vi "Lab Panel V4.86.vi"() -> ()   [LabVIEW 2013] (continued)
                      frame True {
                      }
                    }
                    n1931 = Unbundle By Name(w3326) -> ("1  (A) cal"=w3319:dbl, "1 (V) cal"=w3318:dbl, "1 (PF) cal"=w3317:dbl, "2 (A) cal"=w3316:dbl, "2 (V) cal"=w3315:dbl, "2 (PF) cal"=w3314:dbl)  [unwired: 4 out]
                    n1932 = Multiply(x=w3325, y=w3319) -> (x*y=w3312:dbl)
                    n1933 = Multiply(x=w3324, y=w3318) -> (x*y=w3311:dbl)
                    n1934 = Multiply(x=w3323, y=w3317) -> (x*y=w3310:dbl)
                    n1935 = Multiply(x=w3322, y=w3316) -> (x*y=w3308:dbl)
                    n1936 = Multiply(x=w3321, y=w3315) -> (x*y=w3307:dbl)
                    n1937 = Multiply(x=w3320, y=w3314) -> (x*y=w3306:dbl)
                    n1938 = local read "SIG LAB04-1"() -> (w3313:T2)
                    n1939 = local read "SIG LAB04-2"() -> (w3309:T2)
                    n1940 = Bundle By Name(cluster=w3313, "AMPS"=w3312, "VOLTS"=w3311, "PF"=w3310) -> (w3302:T2)
                    n1941 = Bundle By Name(cluster=w3309, "AMPS"=w3308, "VOLTS"=w3307, "PF"=w3306) -> (w3301:T2)
                    n1942 = global write "Global display 1.vi" "SIG LAB04-2"(w3301) -> ()
                    n1943 = global write "Global display 1.vi" "SIG LAB04-1"(w3302) -> ()
                    n1944 = local write "SIG LAB04-2"(w3301) -> ()
                    n1945 = local write "SIG LAB04-1"(w3302) -> ()
                  }
                  frame #5 {
                    n1946 = Unbundle By Name(w3334) -> ("LAB05-1 (A)"=w3353:dbl, "LAB05-1 (V)"=w3333:dbl, "LAB05-1 (PF)"=w3352:dbl, "LAB05-2 (A)"=w3351:dbl, "LAB05-2 (V)"=w3350:dbl, "LAB05-2 (PF)"=w3349:dbl)
                    n1947 = case shown="False" w3332 {
                      tunnel: [w3355 w3356] -> w3354
                      tunnel: w3331 -> [_ w3356]
                      frame False {
                        n1948 = local read "CAL LAB05"() -> (w3355:T12)
                      }
                      frame True {
                      }
                    }
                    n1949 = Unbundle By Name(w3354) -> ("1  (A) cal"=w3348:dbl, "1 (V) cal"=w3347:dbl, "1 (PF) cal"=w3346:dbl, "2 (A) cal"=w3345:dbl, "2 (V) cal"=w3344:dbl, "2 (PF) cal"=w3343:dbl)  [unwired: 4 out]
                    n1950 = Multiply(x=w3353, y=w3348) -> (x*y=w3341:dbl)
                    n1951 = Multiply(x=w3333, y=w3347) -> (x*y=w3340:dbl)
                    n1952 = Multiply(x=w3352, y=w3346) -> (x*y=w3339:dbl)
                    n1953 = Multiply(x=w3351, y=w3345) -> (x*y=w3337:dbl)
                    n1954 = Multiply(x=w3350, y=w3344) -> (x*y=w3336:dbl)
                    n1955 = Multiply(x=w3349, y=w3343) -> (x*y=w3335:dbl)
                    n1956 = local read "SIG LAB05-1"() -> (w3342:T2)
                    n1957 = local read "SIG LAB05-2"() -> (w3338:T2)
                    n1958 = Bundle By Name(cluster=w3342, "AMPS"=w3341, "VOLTS"=w3340, "PF"=w3339) -> (w3330:T2)
                    n1959 = Bundle By Name(cluster=w3338, "AMPS"=w3337, "VOLTS"=w3336, "PF"=w3335) -> (w3329:T2)
                    n1960 = global write "Global display 1.vi" "SIG LAB05-1"(w3330) -> ()
                    n1961 = global write "Global display 1.vi" "SIG LAB05-2"(w3329) -> ()
                    n1962 = local write "SIG LAB05-2"(w3329) -> ()
                    n1963 = local write "SIG LAB05-1"(w3330) -> ()
                  }
                }
              }
            }
          }
          frame #12 {
            # "save test data to file"
            n1964 = Get Date/Time In Seconds() -> (seconds since 1Jan1904=w3357:timestamp)
            "File Time Stamp" <- w3357
            n1965 = local read "on loops"() -> (w3376:dbl)
            n1966 = local read "jig cycle"() -> (w3373:dbl)
            n1967 = Format Date/Time String(time format string (%c)="%H:%M%:%S", seconds (now)=w3357) -> (date/time string=w3361:string)  [unwired: 1 in]
            n1968 = Add(x=w3376, y=2) -> (x+y=w3374:dbl)
            n1969 = Build Array(w3361) -> (w3360:string[])
            n1970 = Equal?(x=w3373, y=1) -> (x = y?=w3359:bool)
            n1971 = Equal?(x=w3373, y=w3374) -> (x = y?=w3358:bool)
            n1972 = stacked-sequence {
              tunnel: w3372 -> [w3382 _ _ _ _ _ _ _ _ _]
              tunnel: w3371 -> [_ w3458 _ _ _ _ _ _ _ _]
              tunnel: w3370 -> [_ _ w3538 _ _ _ _ _ _ _]
              tunnel: w3369 -> [_ _ _ w3618 _ _ _ _ _ _]
              tunnel: w3368 -> [_ _ _ _ w3698 _ _ _ _ _]
              tunnel: w3367 -> [_ _ _ _ _ w3778 _ _ _ _]
              tunnel: w3366 -> [_ _ _ _ _ _ w3858 _ _ _]
              tunnel: w3365 -> [_ _ _ _ _ _ _ w3938 _ _]
              tunnel: w3364 -> [_ _ _ _ _ _ _ _ w4018 _]
              tunnel: w3363 -> [_ _ _ _ _ _ _ _ _ w4098]
              tunnel: w3360 -> [w3381 w3462 w3542 w3622 w3702 w3782 w3862 w3942 w4022 w4102]
              tunnel: w3359 -> [w3380 w3461 w3541 w3621 w3701 w3781 w3861 w3941 w4021 w4101]
              tunnel: w3358 -> [w3379 w3460 w3540 w3620 w3700 w3780 w3860 w3940 w4020 w4100]
              tunnel: w3357 -> [w3378 w3459 w3539 w3619 w3699 w3779 w3859 w3939 w4019 w4099]
              frame #0 {
                n1973 = case shown="True" w3382 {
                  tunnel: w3381 -> [_ w3387]
                  tunnel: w3380 -> [_ w3386]
                  tunnel: w3379 -> [_ w3384]
                  tunnel: w3378 -> [_ w3383]
                  frame False {
                  }
                  frame True {
                    n1974 = local read "DISP LAB01-1"() -> (w3388:T4)
                    n1975 = local read "SIG LAB01-1"() -> (w3389:T2)
                    n1976 = local read "ON L01-1"() -> (w3385:cluster{"amps":dbl, "volts":dbl, "pf":dbl})
                    n1977 = Unbundle(w3389) -> ("AMPS"=w3395:dbl, "VOLTS"=w3393:dbl, "PF"=w3392:dbl, "Tmp Live"=w3391:dbl, "Tmp Neut"=w3394:dbl)
                    n1978 = Unbundle(w3388) -> ("CYCLE"=w3390:dbl)  [unwired: 2 out]
                    n1979 = stacked-sequence {
                      tunnel: w3395 -> [w3399 w3418]
                      tunnel: w3394 -> [_ w3417]
                      tunnel: w3393 -> [w3398 w3416]
                      tunnel: w3392 -> [w3397 w3415]
                      tunnel: w3391 -> [_ w3414]
                      tunnel: w3390 -> [_ w3413]
                      tunnel: w3387 -> [_ w3412]
                      tunnel: w3386 -> [w3400 _]
                      tunnel: w3385 -> [w3396 w3410]
                      tunnel: w3384 -> [_ w3411]
                      tunnel: w3383 -> [_ w3406]
                      frame #0 {
                        n1980 = case shown="True" w3400 {
                          tunnel: w3399 -> [_ w3405]
                          tunnel: w3398 -> [_ w3404]
                          tunnel: w3397 -> [_ w3403]
                          tunnel: w3396 -> [_ w3401]
                          frame False {
                          }
                          frame True {
                            n1981 = Bundle(cluster=w3401, "amps"=w3405, "volts"=w3404, "pf"=w3403) -> (w3402:cluster{"amps":dbl, "volts":dbl, "pf":dbl})
                            n1982 = local write "ON L01-1"(w3402) -> ()
                          }
                        }
                      }
                      frame #1 {
                        n1983 = Unbundle(w3410) -> ("amps"=w3409:dbl, "volts"=w3408:dbl, "pf"=w3407:dbl)
                        n1984 = case shown="True" w3411 {
                          tunnel: w3418 -> [_ w3419]
                          tunnel: w3417 -> [_ w3457]
                          tunnel: w3416 -> [_ _]
                          tunnel: w3415 -> [_ _]
                          tunnel: w3414 -> [_ w3456]
                          tunnel: w3413 -> [_ w3455]
                          tunnel: w3412 -> [_ w3423]
                          tunnel: w3409 -> [_ w3420]
                          tunnel: w3408 -> [_ w3452]
                          tunnel: w3407 -> [_ w3451]
                          tunnel: w3406 -> [_ w3421]
                          frame False {
                          }
                          frame True {
                            n1985 = local read "TDMS LAB01-1"() -> (w3454:refnum<k34>)
                            n1986 = Build Array(w3452) -> (w3448:dbl[])
                            n1987 = Build Array(w3451) -> (w3447:dbl[])
                            n1988 = Build Array(w3456) -> (w3446:dbl[])
                            n1989 = Build Array(w3457) -> (w3445:dbl[])
                            n1990 = Build Array(w3420) -> (w3450:dbl[])
                            n1991 = Build Array(w3419) -> (w3449:dbl[])
                            n1992 = Build Array(w3455) -> (w3444:dbl[])
                            n1993 = Build Array("AMPS ON", "AMPS OFF", "VOLTS", "PF", "TEMP Live", "TEMP Neut", "CYCLE") -> (w3428:string[])
                            n1994 = Bundle By Name("Y"=w3450, "t0"=w3421) -> (w3443:waveform(dbl))  [unwired: 1 in]
                            n1995 = Bundle By Name("Y"=w3449, "t0"=w3421) -> (w3442:waveform(dbl))  [unwired: 1 in]
                            n1996 = Bundle By Name("Y"=w3448, "t0"=w3421) -> (w3441:waveform(dbl))  [unwired: 1 in]
                            n1997 = Bundle By Name("Y"=w3447, "t0"=w3421) -> (w3440:waveform(dbl))  [unwired: 1 in]
                            n1998 = Bundle By Name("Y"=w3446, "t0"=w3421) -> (w3439:waveform(dbl))  [unwired: 1 in]
                            n1999 = Bundle By Name("Y"=w3445, "t0"=w3421) -> (w3438:waveform(dbl))  [unwired: 1 in]
                            n2000 = Bundle By Name("Y"=w3444, "t0"=w3421) -> (w3437:waveform(dbl))  [unwired: 1 in]
                            n2001 = Build Array(w3443, w3442, w3441, w3440, w3439, w3438, w3437) -> (w3436:waveform(dbl)[])
                            n2002 = TDMS Write(0:w3454, 5:"TEST VALUES", 7:w3428, 9:w3436) -> (4:w3427:refnum<k34>, 6:w3426:string, 15:w3425:errorcluster)  [unwired: 2 in, 1 out]
                            n2003 = TDMS Write(0:w3427, 5:w3426, 7:"TIME", 9:w3423, 11:w3425) -> (15:w3422:errorcluster)  [unwired: 1 in, 3 out]
                            n2004 = local write "data file error"(w3422) -> ()
                          }
                        }
                      }
                    }
                  }
                }
              }
              frame #1 {
                n2005 = case shown="True" w3458 {
                  tunnel: w3462 -> [_ w3467]
                  tunnel: w3461 -> [_ w3466]
                  tunnel: w3460 -> [_ w3464]
                  tunnel: w3459 -> [_ w3463]
                  frame False {
                  }
                  frame True {
                    n2006 = local read "DISP LAB01-2"() -> (w3468:T4)
                    n2007 = local read "SIG LAB01-2"() -> (w3469:T2)
                    n2008 = local read "ON L01-2"() -> (w3465:cluster{"amps":dbl, "volts":dbl, "pf":dbl})
                    n2009 = Unbundle(w3469) -> ("AMPS"=w3475:dbl, "VOLTS"=w3473:dbl, "PF"=w3472:dbl, "Tmp Live"=w3471:dbl, "Tmp Neut"=w3474:dbl)
                    n2010 = Unbundle(w3468) -> ("CYCLE"=w3470:dbl)  [unwired: 2 out]
                    n2011 = stacked-sequence {
                      tunnel: w3475 -> [w3479 w3498]
                      tunnel: w3474 -> [_ w3497]
                      tunnel: w3473 -> [w3478 w3496]
                      tunnel: w3472 -> [w3477 w3495]
                      tunnel: w3471 -> [_ w3494]
                      tunnel: w3470 -> [_ w3493]
                      tunnel: w3467 -> [_ w3492]
                      tunnel: w3466 -> [w3480 _]
                      tunnel: w3465 -> [w3476 w3490]
                      tunnel: w3464 -> [_ w3491]
                      tunnel: w3463 -> [_ w3486]
                      frame #0 {
                        n2012 = case shown="True" w3480 {
                          tunnel: w3479 -> [_ w3485]
                          tunnel: w3478 -> [_ w3484]
                          tunnel: w3477 -> [_ w3483]
                          tunnel: w3476 -> [_ w3481]
                          frame False {
                          }
                          frame True {
                            n2013 = Bundle(cluster=w3481, "amps"=w3485, "volts"=w3484, "pf"=w3483) -> (w3482:cluster{"amps":dbl, "volts":dbl, "pf":dbl})
                            n2014 = local write "ON L01-2"(w3482) -> ()
                          }
                        }
                      }
                      frame #1 {
                        n2015 = Unbundle(w3490) -> ("amps"=w3489:dbl, "volts"=w3488:dbl, "pf"=w3487:dbl)
                        n2016 = case shown="True" w3491 {
                          tunnel: w3498 -> [_ w3530]
                          tunnel: w3497 -> [_ w3537]
                          tunnel: w3496 -> [_ _]
                          tunnel: w3495 -> [_ _]
                          tunnel: w3494 -> [_ w3536]
                          tunnel: w3493 -> [_ w3535]
                          tunnel: w3492 -> [_ w3500]
                          tunnel: w3489 -> [_ w3532]
                          tunnel: w3488 -> [_ w3531]
                          tunnel: w3487 -> [_ w3529]
                          tunnel: w3486 -> [_ w3521]
                          frame False {
                          }
                          frame True {
                            n2017 = local read "TDMS LAB01-2"() -> (w3534:refnum<k34>)
                            n2018 = Build Array(w3531) -> (w3526:dbl[])
                            n2019 = Build Array(w3529) -> (w3525:dbl[])
                            n2020 = Build Array(w3536) -> (w3524:dbl[])
                            n2021 = Build Array(w3537) -> (w3523:dbl[])
                            n2022 = Build Array(w3532) -> (w3528:dbl[])
                            n2023 = Build Array(w3530) -> (w3527:dbl[])
                            n2024 = Build Array(w3535) -> (w3522:dbl[])
                            n2025 = Build Array("AMPS ON", "AMPS OFF", "VOLTS", "PF", "TEMP Live", "TEMP Neut", "CYCLE") -> (w3505:string[])
                            n2026 = Bundle By Name("Y"=w3528, "t0"=w3521) -> (w3520:waveform(dbl))  [unwired: 1 in]
                            n2027 = Bundle By Name("Y"=w3527, "t0"=w3521) -> (w3519:waveform(dbl))  [unwired: 1 in]
                            n2028 = Bundle By Name("Y"=w3526, "t0"=w3521) -> (w3518:waveform(dbl))  [unwired: 1 in]
                            n2029 = Bundle By Name("Y"=w3525, "t0"=w3521) -> (w3517:waveform(dbl))  [unwired: 1 in]
                            n2030 = Bundle By Name("Y"=w3524, "t0"=w3521) -> (w3516:waveform(dbl))  [unwired: 1 in]
                            n2031 = Bundle By Name("Y"=w3523, "t0"=w3521) -> (w3515:waveform(dbl))  [unwired: 1 in]
                            n2032 = Bundle By Name("Y"=w3522, "t0"=w3521) -> (w3514:waveform(dbl))  [unwired: 1 in]
                            n2033 = Build Array(w3520, w3519, w3518, w3517, w3516, w3515, w3514) -> (w3513:waveform(dbl)[])
                            n2034 = TDMS Write(0:w3534, 5:"TEST VALUES", 7:w3505, 9:w3513) -> (4:w3504:refnum<k34>, 6:w3503:string, 15:w3502:errorcluster)  [unwired: 2 in, 1 out]
                            n2035 = TDMS Write(0:w3504, 5:w3503, 7:"TIME", 9:w3500, 11:w3502) -> (15:w3499:errorcluster)  [unwired: 1 in, 3 out]
                            n2036 = local write "data file error"(w3499) -> ()
                          }
                        }
                      }
                    }
                  }
                }
              }
              frame #2 {
                n2037 = case shown="True" w3538 {
                  tunnel: w3542 -> [_ w3547]
                  tunnel: w3541 -> [_ w3546]
                  tunnel: w3540 -> [_ w3544]
                  tunnel: w3539 -> [_ w3543]
                  frame False {
                  }
                  frame True {
                    n2038 = local read "DISP LAB02-1"() -> (w3548:T4)
                    n2039 = local read "SIG LAB02-1"() -> (w3549:T2)
                    n2040 = local read "ON L02-1"() -> (w3545:cluster{"amps":dbl, "volts":dbl, "pf":dbl})
                    n2041 = Unbundle(w3549) -> ("AMPS"=w3555:dbl, "VOLTS"=w3553:dbl, "PF"=w3552:dbl, "Tmp Live"=w3551:dbl, "Tmp Neut"=w3554:dbl)
                    n2042 = Unbundle(w3548) -> ("CYCLE"=w3550:dbl)  [unwired: 2 out]
                    n2043 = stacked-sequence {
                      tunnel: w3555 -> [w3559 w3578]
                      tunnel: w3554 -> [_ w3577]
                      tunnel: w3553 -> [w3558 w3576]
                      tunnel: w3552 -> [w3557 w3575]
                      tunnel: w3551 -> [_ w3574]
                      tunnel: w3550 -> [_ w3573]
                      tunnel: w3547 -> [_ w3572]
                      tunnel: w3546 -> [w3560 _]
                      tunnel: w3545 -> [w3556 w3570]
                      tunnel: w3544 -> [_ w3571]
                      tunnel: w3543 -> [_ w3566]
                      frame #0 {
                        n2044 = case shown="True" w3560 {
                          tunnel: w3559 -> [_ w3565]
                          tunnel: w3558 -> [_ w3564]
                          tunnel: w3557 -> [_ w3563]
                          tunnel: w3556 -> [_ w3561]
                          frame False {
                          }
                          frame True {
                            n2045 = Bundle(cluster=w3561, "amps"=w3565, "volts"=w3564, "pf"=w3563) -> (w3562:cluster{"amps":dbl, "volts":dbl, "pf":dbl})
                            n2046 = local write "ON L02-1"(w3562) -> ()
                          }
                        }
                      }
                      frame #1 {
                        n2047 = Unbundle(w3570) -> ("amps"=w3569:dbl, "volts"=w3568:dbl, "pf"=w3567:dbl)
                        n2048 = case shown="True" w3571 {
                          tunnel: w3578 -> [_ w3610]
                          tunnel: w3577 -> [_ w3617]
                          tunnel: w3576 -> [_ _]
                          tunnel: w3575 -> [_ _]
                          tunnel: w3574 -> [_ w3616]
                          tunnel: w3573 -> [_ w3615]
                          tunnel: w3572 -> [_ w3580]
                          tunnel: w3569 -> [_ w3612]
                          tunnel: w3568 -> [_ w3611]
                          tunnel: w3567 -> [_ w3609]
                          tunnel: w3566 -> [_ w3601]
                          frame False {
                          }
                          frame True {
                            n2049 = local read "TDMS LAB02-1"() -> (w3614:refnum<k34>)
                            n2050 = Build Array(w3611) -> (w3606:dbl[])
                            n2051 = Build Array(w3609) -> (w3605:dbl[])
                            n2052 = Build Array(w3616) -> (w3604:dbl[])
                            n2053 = Build Array(w3617) -> (w3603:dbl[])
                            n2054 = Build Array(w3612) -> (w3608:dbl[])
                            n2055 = Build Array(w3610) -> (w3607:dbl[])
                            n2056 = Build Array(w3615) -> (w3602:dbl[])
                            n2057 = Build Array("AMPS ON", "AMPS OFF", "VOLTS", "PF", "TEMP Live", "TEMP Neut", "CYCLE") -> (w3585:string[])
                            n2058 = Bundle By Name("Y"=w3608, "t0"=w3601) -> (w3600:waveform(dbl))  [unwired: 1 in]
                            n2059 = Bundle By Name("Y"=w3607, "t0"=w3601) -> (w3599:waveform(dbl))  [unwired: 1 in]
                            n2060 = Bundle By Name("Y"=w3606, "t0"=w3601) -> (w3598:waveform(dbl))  [unwired: 1 in]
                            n2061 = Bundle By Name("Y"=w3605, "t0"=w3601) -> (w3597:waveform(dbl))  [unwired: 1 in]
                            n2062 = Bundle By Name("Y"=w3604, "t0"=w3601) -> (w3596:waveform(dbl))  [unwired: 1 in]
                            n2063 = Bundle By Name("Y"=w3603, "t0"=w3601) -> (w3595:waveform(dbl))  [unwired: 1 in]
                            n2064 = Bundle By Name("Y"=w3602, "t0"=w3601) -> (w3594:waveform(dbl))  [unwired: 1 in]
                            n2065 = Build Array(w3600, w3599, w3598, w3597, w3596, w3595, w3594) -> (w3593:waveform(dbl)[])
                            n2066 = TDMS Write(0:w3614, 5:"TEST VALUES", 7:w3585, 9:w3593) -> (4:w3584:refnum<k34>, 6:w3583:string, 15:w3582:errorcluster)  [unwired: 2 in, 1 out]
                            n2067 = TDMS Write(0:w3584, 5:w3583, 7:"TIME", 9:w3580, 11:w3582) -> (15:w3579:errorcluster)  [unwired: 1 in, 3 out]
                            n2068 = local write "data file error"(w3579) -> ()
                          }
                        }
                      }
                    }
                  }
                }
              }
              frame #3 {
                n2069 = case shown="True" w3618 {
                  tunnel: w3622 -> [_ w3627]
                  tunnel: w3621 -> [_ w3626]
                  tunnel: w3620 -> [_ w3624]
                  tunnel: w3619 -> [_ w3623]
                  frame False {
                  }
                  frame True {
                    n2070 = local read "DISP LAB02-2"() -> (w3628:T4)
                    n2071 = local read "SIG LAB02-2"() -> (w3629:T2)
                    n2072 = local read "ON L02-2"() -> (w3625:cluster{"amps":dbl, "volts":dbl, "pf":dbl})
                    n2073 = Unbundle(w3629) -> ("AMPS"=w3635:dbl, "VOLTS"=w3633:dbl, "PF"=w3632:dbl, "Tmp Live"=w3631:dbl, "Tmp Neut"=w3634:dbl)
                    n2074 = Unbundle(w3628) -> ("CYCLE"=w3630:dbl)  [unwired: 2 out]
                    n2075 = stacked-sequence {
                      tunnel: w3635 -> [w3639 w3658]
                      tunnel: w3634 -> [_ w3657]
                      tunnel: w3633 -> [w3638 w3656]
                      tunnel: w3632 -> [w3637 w3655]
                      tunnel: w3631 -> [_ w3654]
                      tunnel: w3630 -> [_ w3653]
                      tunnel: w3627 -> [_ w3652]
                      tunnel: w3626 -> [w3640 _]
                      tunnel: w3625 -> [w3636 w3650]
                      tunnel: w3624 -> [_ w3651]
                      tunnel: w3623 -> [_ w3646]
                      frame #0 {
                        n2076 = case shown="True" w3640 {
                          tunnel: w3639 -> [_ w3645]
                          tunnel: w3638 -> [_ w3644]
                          tunnel: w3637 -> [_ w3643]
                          tunnel: w3636 -> [_ w3641]
                          frame False {
                          }
                          frame True {
                            n2077 = Bundle(cluster=w3641, "amps"=w3645, "volts"=w3644, "pf"=w3643) -> (w3642:cluster{"amps":dbl, "volts":dbl, "pf":dbl})
                            n2078 = local write "ON L02-2"(w3642) -> ()
                          }
                        }
                      }
                      frame #1 {
                        n2079 = Unbundle(w3650) -> ("amps"=w3649:dbl, "volts"=w3648:dbl, "pf"=w3647:dbl)
                        n2080 = case shown="True" w3651 {
                          tunnel: w3658 -> [_ w3690]
                          tunnel: w3657 -> [_ w3697]
                          tunnel: w3656 -> [_ _]
                          tunnel: w3655 -> [_ _]
                          tunnel: w3654 -> [_ w3696]
                          tunnel: w3653 -> [_ w3695]
                          tunnel: w3652 -> [_ w3660]
                          tunnel: w3649 -> [_ w3692]
                          tunnel: w3648 -> [_ w3691]
                          tunnel: w3647 -> [_ w3689]
                          tunnel: w3646 -> [_ w3681]
                          frame False {
                          }
                          frame True {
                            n2081 = local read "TDMS LAB02-2"() -> (w3694:refnum<k34>)
                            n2082 = Build Array(w3691) -> (w3686:dbl[])
                            n2083 = Build Array(w3689) -> (w3685:dbl[])
                            n2084 = Build Array(w3696) -> (w3684:dbl[])
                            n2085 = Build Array(w3697) -> (w3683:dbl[])
                            n2086 = Build Array(w3692) -> (w3688:dbl[])
                            n2087 = Build Array(w3690) -> (w3687:dbl[])
                            n2088 = Build Array(w3695) -> (w3682:dbl[])
                            n2089 = Build Array("AMPS ON", "AMPS OFF", "VOLTS", "PF", "TEMP Live", "TEMP Neut", "CYCLE") -> (w3665:string[])
                            n2090 = Bundle By Name("Y"=w3688, "t0"=w3681) -> (w3680:waveform(dbl))  [unwired: 1 in]
                            n2091 = Bundle By Name("Y"=w3687, "t0"=w3681) -> (w3679:waveform(dbl))  [unwired: 1 in]
                            n2092 = Bundle By Name("Y"=w3686, "t0"=w3681) -> (w3678:waveform(dbl))  [unwired: 1 in]
                            n2093 = Bundle By Name("Y"=w3685, "t0"=w3681) -> (w3677:waveform(dbl))  [unwired: 1 in]
                            n2094 = Bundle By Name("Y"=w3684, "t0"=w3681) -> (w3676:waveform(dbl))  [unwired: 1 in]
                            n2095 = Bundle By Name("Y"=w3683, "t0"=w3681) -> (w3675:waveform(dbl))  [unwired: 1 in]
                            n2096 = Bundle By Name("Y"=w3682, "t0"=w3681) -> (w3674:waveform(dbl))  [unwired: 1 in]
                            n2097 = Build Array(w3680, w3679, w3678, w3677, w3676, w3675, w3674) -> (w3673:waveform(dbl)[])
                            n2098 = TDMS Write(0:w3694, 5:"TEST VALUES", 7:w3665, 9:w3673) -> (4:w3664:refnum<k34>, 6:w3663:string, 15:w3662:errorcluster)  [unwired: 2 in, 1 out]
                            n2099 = TDMS Write(0:w3664, 5:w3663, 7:"TIME", 9:w3660, 11:w3662) -> (15:w3659:errorcluster)  [unwired: 1 in, 3 out]
                            n2100 = local write "data file error"(w3659) -> ()
                          }
                        }
                      }
                    }
                  }
                }
              }
              frame #4 {
                n2101 = case shown="True" w3698 {
                  tunnel: w3702 -> [_ w3707]
                  tunnel: w3701 -> [_ w3706]
                  tunnel: w3700 -> [_ w3704]
                  tunnel: w3699 -> [_ w3703]
                  frame False {
                  }
                  frame True {
                    n2102 = local read "DISP LAB03-1"() -> (w3708:T4)
                    n2103 = local read "SIG LAB03-1"() -> (w3709:T2)
                    n2104 = local read "ON L03-1"() -> (w3705:cluster{"amps":dbl, "volts":dbl, "pf":dbl})
                    n2105 = Unbundle(w3709) -> ("AMPS"=w3715:dbl, "VOLTS"=w3713:dbl, "PF"=w3712:dbl, "Tmp Live"=w3711:dbl, "Tmp Neut"=w3714:dbl)
                    n2106 = Unbundle(w3708) -> ("CYCLE"=w3710:dbl)  [unwired: 2 out]
                    n2107 = stacked-sequence {
                      tunnel: w3715 -> [w3719 w3738]
                      tunnel: w3714 -> [_ w3737]
                      tunnel: w3713 -> [w3718 w3736]
                      tunnel: w3712 -> [w3717 w3735]
                      tunnel: w3711 -> [_ w3734]
                      tunnel: w3710 -> [_ w3733]
                      tunnel: w3707 -> [_ w3732]
                      tunnel: w3706 -> [w3720 _]
                      tunnel: w3705 -> [w3716 w3730]
                      tunnel: w3704 -> [_ w3731]
                      tunnel: w3703 -> [_ w3726]
                      frame #0 {
                        n2108 = case shown="True" w3720 {
                          tunnel: w3719 -> [_ w3725]
                          tunnel: w3718 -> [_ w3724]
                          tunnel: w3717 -> [_ w3723]
                          tunnel: w3716 -> [_ w3721]
                          frame False {
                          }
                          frame True {
                            n2109 = Bundle(cluster=w3721, "amps"=w3725, "volts"=w3724, "pf"=w3723) -> (w3722:cluster{"amps":dbl, "volts":dbl, "pf":dbl})
                            n2110 = local write "ON L03-1"(w3722) -> ()
                          }
                        }
                      }
                      frame #1 {
                        n2111 = Unbundle(w3730) -> ("amps"=w3729:dbl, "volts"=w3728:dbl, "pf"=w3727:dbl)
                        n2112 = case shown="True" w3731 {
                          tunnel: w3738 -> [_ w3770]
                          tunnel: w3737 -> [_ w3777]
                          tunnel: w3736 -> [_ _]
                          tunnel: w3735 -> [_ _]
                          tunnel: w3734 -> [_ w3776]
                          tunnel: w3733 -> [_ w3775]
                          tunnel: w3732 -> [_ w3740]
                          tunnel: w3729 -> [_ w3772]
                          tunnel: w3728 -> [_ w3771]
                          tunnel: w3727 -> [_ w3769]
                          tunnel: w3726 -> [_ w3761]
                          frame False {
                          }
                          frame True {
                            n2113 = local read "TDMS LAB03-1"() -> (w3774:refnum<k34>)
                            n2114 = Build Array(w3771) -> (w3766:dbl[])
                            n2115 = Build Array(w3769) -> (w3765:dbl[])
                            n2116 = Build Array(w3776) -> (w3764:dbl[])
                            n2117 = Build Array(w3777) -> (w3763:dbl[])
                            n2118 = Build Array(w3772) -> (w3768:dbl[])
                            n2119 = Build Array(w3770) -> (w3767:dbl[])
                            n2120 = Build Array(w3775) -> (w3762:dbl[])
                            n2121 = Build Array("AMPS ON", "AMPS OFF", "VOLTS", "PF", "TEMP Live", "TEMP Neut", "CYCLE") -> (w3745:string[])
                            n2122 = Bundle By Name("Y"=w3768, "t0"=w3761) -> (w3760:waveform(dbl))  [unwired: 1 in]
                            n2123 = Bundle By Name("Y"=w3767, "t0"=w3761) -> (w3759:waveform(dbl))  [unwired: 1 in]
                            n2124 = Bundle By Name("Y"=w3766, "t0"=w3761) -> (w3758:waveform(dbl))  [unwired: 1 in]
                            n2125 = Bundle By Name("Y"=w3765, "t0"=w3761) -> (w3757:waveform(dbl))  [unwired: 1 in]
                            n2126 = Bundle By Name("Y"=w3764, "t0"=w3761) -> (w3756:waveform(dbl))  [unwired: 1 in]
                            n2127 = Bundle By Name("Y"=w3763, "t0"=w3761) -> (w3755:waveform(dbl))  [unwired: 1 in]
                            n2128 = Bundle By Name("Y"=w3762, "t0"=w3761) -> (w3754:waveform(dbl))  [unwired: 1 in]
                            n2129 = Build Array(w3760, w3759, w3758, w3757, w3756, w3755, w3754) -> (w3753:waveform(dbl)[])
                            n2130 = TDMS Write(0:w3774, 5:"TEST VALUES", 7:w3745, 9:w3753) -> (4:w3744:refnum<k34>, 6:w3743:string, 15:w3742:errorcluster)  [unwired: 2 in, 1 out]
                            n2131 = TDMS Write(0:w3744, 5:w3743, 7:"TIME", 9:w3740, 11:w3742) -> (15:w3739:errorcluster)  [unwired: 1 in, 3 out]
                            n2132 = local write "data file error"(w3739) -> ()
                          }
                        }
                      }
                    }
                  }
                }
              }
              frame #5 {
                n2133 = case shown="True" w3778 {
                  tunnel: w3782 -> [_ w3787]
                  tunnel: w3781 -> [_ w3786]
                  tunnel: w3780 -> [_ w3784]
                  tunnel: w3779 -> [_ w3783]
                  frame False {
                  }
                  frame True {
                    n2134 = local read "DISP LAB03-2"() -> (w3788:T4)
                    n2135 = local read "SIG LAB03-2"() -> (w3789:T2)
                    n2136 = local read "ON L03-2"() -> (w3785:cluster{"amps":dbl, "volts":dbl, "pf":dbl})
                    n2137 = Unbundle(w3789) -> ("AMPS"=w3795:dbl, "VOLTS"=w3793:dbl, "PF"=w3792:dbl, "Tmp Live"=w3791:dbl, "Tmp Neut"=w3794:dbl)
                    n2138 = Unbundle(w3788) -> ("CYCLE"=w3790:dbl)  [unwired: 2 out]
                    n2139 = stacked-sequence {
                      tunnel: w3795 -> [w3799 w3818]
                      tunnel: w3794 -> [_ w3817]
                      tunnel: w3793 -> [w3798 w3816]
                      tunnel: w3792 -> [w3797 w3815]
                      tunnel: w3791 -> [_ w3814]
                      tunnel: w3790 -> [_ w3813]
                      tunnel: w3787 -> [_ w3812]
                      tunnel: w3786 -> [w3800 _]
                      tunnel: w3785 -> [w3796 w3810]
                      tunnel: w3784 -> [_ w3811]
                      tunnel: w3783 -> [_ w3806]
                      frame #0 {
                        n2140 = case shown="True" w3800 {
                          tunnel: w3799 -> [_ w3805]
                          tunnel: w3798 -> [_ w3804]
                          tunnel: w3797 -> [_ w3803]
                          tunnel: w3796 -> [_ w3801]
                          frame False {
                          }
                          frame True {
                            n2141 = Bundle(cluster=w3801, "amps"=w3805, "volts"=w3804, "pf"=w3803) -> (w3802:cluster{"amps":dbl, "volts":dbl, "pf":dbl})
                            n2142 = local write "ON L03-2"(w3802) -> ()
                          }
                        }
                      }
                      frame #1 {
                        n2143 = Unbundle(w3810) -> ("amps"=w3809:dbl, "volts"=w3808:dbl, "pf"=w3807:dbl)
                        n2144 = case shown="True" w3811 {
                          tunnel: w3818 -> [_ w3850]
                          tunnel: w3817 -> [_ w3857]
                          tunnel: w3816 -> [_ _]
                          tunnel: w3815 -> [_ _]
                          tunnel: w3814 -> [_ w3856]
                          tunnel: w3813 -> [_ w3855]
                          tunnel: w3812 -> [_ w3820]
                          tunnel: w3809 -> [_ w3852]
                          tunnel: w3808 -> [_ w3851]
                          tunnel: w3807 -> [_ w3849]
                          tunnel: w3806 -> [_ w3841]
                          frame False {
                          }
                          frame True {
                            n2145 = local read "TDMS LAB03-2"() -> (w3854:refnum<k34>)
                            n2146 = Build Array(w3851) -> (w3846:dbl[])
                            n2147 = Build Array(w3849) -> (w3845:dbl[])
                            n2148 = Build Array(w3856) -> (w3844:dbl[])
                            n2149 = Build Array(w3857) -> (w3843:dbl[])
                            n2150 = Build Array(w3852) -> (w3848:dbl[])
                            n2151 = Build Array(w3850) -> (w3847:dbl[])
                            n2152 = Build Array(w3855) -> (w3842:dbl[])
                            n2153 = Build Array("AMPS ON", "AMPS OFF", "VOLTS", "PF", "TEMP Live", "TEMP Neut", "CYCLE") -> (w3825:string[])
                            n2154 = Bundle By Name("Y"=w3848, "t0"=w3841) -> (w3840:waveform(dbl))  [unwired: 1 in]
                            n2155 = Bundle By Name("Y"=w3847, "t0"=w3841) -> (w3839:waveform(dbl))  [unwired: 1 in]
                            n2156 = Bundle By Name("Y"=w3846, "t0"=w3841) -> (w3838:waveform(dbl))  [unwired: 1 in]
                            n2157 = Bundle By Name("Y"=w3845, "t0"=w3841) -> (w3837:waveform(dbl))  [unwired: 1 in]
                            n2158 = Bundle By Name("Y"=w3844, "t0"=w3841) -> (w3836:waveform(dbl))  [unwired: 1 in]
                            n2159 = Bundle By Name("Y"=w3843, "t0"=w3841) -> (w3835:waveform(dbl))  [unwired: 1 in]
                            n2160 = Bundle By Name("Y"=w3842, "t0"=w3841) -> (w3834:waveform(dbl))  [unwired: 1 in]
                            n2161 = Build Array(w3840, w3839, w3838, w3837, w3836, w3835, w3834) -> (w3833:waveform(dbl)[])
                            n2162 = TDMS Write(0:w3854, 5:"TEST VALUES", 7:w3825, 9:w3833) -> (4:w3824:refnum<k34>, 6:w3823:string, 15:w3822:errorcluster)  [unwired: 2 in, 1 out]
                            n2163 = TDMS Write(0:w3824, 5:w3823, 7:"TIME", 9:w3820, 11:w3822) -> (15:w3819:errorcluster)  [unwired: 1 in, 3 out]
                            n2164 = local write "data file error"(w3819) -> ()
                          }
                        }
                      }
                    }
                  }
                }
              }
              frame #6 {
                n2165 = case shown="True" w3858 {
                  tunnel: w3862 -> [_ w3867]
                  tunnel: w3861 -> [_ w3866]
                  tunnel: w3860 -> [_ w3864]
                  tunnel: w3859 -> [_ w3863]
                  frame False {
                  }
                  frame True {
                    n2166 = local read "DISP LAB04-1"() -> (w3868:T4)
                    n2167 = local read "SIG LAB04-1"() -> (w3869:T2)
                    n2168 = local read "ON L04-1"() -> (w3865:cluster{"amps":dbl, "volts":dbl, "pf":dbl})
                    n2169 = Unbundle(w3869) -> ("AMPS"=w3875:dbl, "VOLTS"=w3873:dbl, "PF"=w3872:dbl, "Tmp Live"=w3871:dbl, "Tmp Neut"=w3874:dbl)
                    n2170 = Unbundle(w3868) -> ("CYCLE"=w3870:dbl)  [unwired: 2 out]
                    n2171 = stacked-sequence {
                      tunnel: w3875 -> [w3879 w3898]
                      tunnel: w3874 -> [_ w3897]
                      tunnel: w3873 -> [w3878 w3896]
                      tunnel: w3872 -> [w3877 w3895]
                      tunnel: w3871 -> [_ w3894]
                      tunnel: w3870 -> [_ w3893]
                      tunnel: w3867 -> [_ w3892]
                      tunnel: w3866 -> [w3880 _]
                      tunnel: w3865 -> [w3876 w3890]
                      tunnel: w3864 -> [_ w3891]
                      tunnel: w3863 -> [_ w3886]
                      frame #0 {
                        n2172 = case shown="True" w3880 {
                          tunnel: w3879 -> [_ w3885]
                          tunnel: w3878 -> [_ w3884]
                          tunnel: w3877 -> [_ w3883]
                          tunnel: w3876 -> [_ w3881]
                          frame False {
                          }
                          frame True {
                            n2173 = Bundle(cluster=w3881, "amps"=w3885, "volts"=w3884, "pf"=w3883) -> (w3882:cluster{"amps":dbl, "volts":dbl, "pf":dbl})
                            n2174 = local write "ON L04-1"(w3882) -> ()
                          }
                        }
                      }
                      frame #1 {
                        n2175 = Unbundle(w3890) -> ("amps"=w3889:dbl, "volts"=w3888:dbl, "pf"=w3887:dbl)
                        n2176 = case shown="True" w3891 {
                          tunnel: w3898 -> [_ w3930]
                          tunnel: w3897 -> [_ w3937]
                          tunnel: w3896 -> [_ _]
                          tunnel: w3895 -> [_ _]
                          tunnel: w3894 -> [_ w3936]
                          tunnel: w3893 -> [_ w3935]
                          tunnel: w3892 -> [_ w3900]
                          tunnel: w3889 -> [_ w3932]
                          tunnel: w3888 -> [_ w3931]
                          tunnel: w3887 -> [_ w3929]
                          tunnel: w3886 -> [_ w3921]
                          frame False {
                          }
                          frame True {
                            n2177 = local read "TDMS LAB04-1"() -> (w3934:refnum<k34>)
                            n2178 = Build Array(w3931) -> (w3926:dbl[])
                            n2179 = Build Array(w3929) -> (w3925:dbl[])
                            n2180 = Build Array(w3936) -> (w3924:dbl[])
                            n2181 = Build Array(w3937) -> (w3923:dbl[])
                            n2182 = Build Array(w3932) -> (w3928:dbl[])
                            n2183 = Build Array(w3930) -> (w3927:dbl[])
                            n2184 = Build Array(w3935) -> (w3922:dbl[])
                            n2185 = Build Array("AMPS ON", "AMPS OFF", "VOLTS", "PF", "TEMP Live", "TEMP Neut", "CYCLE") -> (w3905:string[])
                            n2186 = Bundle By Name("Y"=w3928, "t0"=w3921) -> (w3920:waveform(dbl))  [unwired: 1 in]
                            n2187 = Bundle By Name("Y"=w3927, "t0"=w3921) -> (w3919:waveform(dbl))  [unwired: 1 in]
                            n2188 = Bundle By Name("Y"=w3926, "t0"=w3921) -> (w3918:waveform(dbl))  [unwired: 1 in]
                            n2189 = Bundle By Name("Y"=w3925, "t0"=w3921) -> (w3917:waveform(dbl))  [unwired: 1 in]
                            n2190 = Bundle By Name("Y"=w3924, "t0"=w3921) -> (w3916:waveform(dbl))  [unwired: 1 in]
                            n2191 = Bundle By Name("Y"=w3923, "t0"=w3921) -> (w3915:waveform(dbl))  [unwired: 1 in]
                            n2192 = Bundle By Name("Y"=w3922, "t0"=w3921) -> (w3914:waveform(dbl))  [unwired: 1 in]
                            n2193 = Build Array(w3920, w3919, w3918, w3917, w3916, w3915, w3914) -> (w3913:waveform(dbl)[])
                            n2194 = TDMS Write(0:w3934, 5:"TEST VALUES", 7:w3905, 9:w3913) -> (4:w3904:refnum<k34>, 6:w3903:string, 15:w3902:errorcluster)  [unwired: 2 in, 1 out]
                            n2195 = TDMS Write(0:w3904, 5:w3903, 7:"TIME", 9:w3900, 11:w3902) -> (15:w3899:errorcluster)  [unwired: 1 in, 3 out]
                            n2196 = local write "data file error"(w3899) -> ()
                          }
                        }
                      }
                    }
                  }
                }
              }
              frame #7 {
                n2197 = case shown="True" w3938 {
                  tunnel: w3942 -> [_ w3947]
                  tunnel: w3941 -> [_ w3946]
                  tunnel: w3940 -> [_ w3944]
                  tunnel: w3939 -> [_ w3943]
                  frame False {
                  }
                  frame True {
                    n2198 = local read "DISP LAB04-2"() -> (w3948:T4)
                    n2199 = local read "SIG LAB04-2"() -> (w3949:T2)
                    n2200 = local read "ON L04-2"() -> (w3945:cluster{"amps":dbl, "volts":dbl, "pf":dbl})
                    n2201 = Unbundle(w3949) -> ("AMPS"=w3955:dbl, "VOLTS"=w3953:dbl, "PF"=w3952:dbl, "Tmp Live"=w3951:dbl, "Tmp Neut"=w3954:dbl)
                    n2202 = Unbundle(w3948) -> ("CYCLE"=w3950:dbl)  [unwired: 2 out]
                    n2203 = stacked-sequence {
                      tunnel: w3955 -> [w3959 w3978]
                      tunnel: w3954 -> [_ w3977]
                      tunnel: w3953 -> [w3958 w3976]
                      tunnel: w3952 -> [w3957 w3975]
                      tunnel: w3951 -> [_ w3974]
                      tunnel: w3950 -> [_ w3973]
                      tunnel: w3947 -> [_ w3972]
                      tunnel: w3946 -> [w3960 _]
                      tunnel: w3945 -> [w3956 w3970]
                      tunnel: w3944 -> [_ w3971]
                      tunnel: w3943 -> [_ w3966]
                      frame #0 {
                        n2204 = case shown="True" w3960 {
                          tunnel: w3959 -> [_ w3965]
                          tunnel: w3958 -> [_ w3964]
                          tunnel: w3957 -> [_ w3963]
                          tunnel: w3956 -> [_ w3961]
                          frame False {
                          }
                          frame True {
                            n2205 = Bundle(cluster=w3961, "amps"=w3965, "volts"=w3964, "pf"=w3963) -> (w3962:cluster{"amps":dbl, "volts":dbl, "pf":dbl})
                            n2206 = local write "ON L04-2"(w3962) -> ()
                          }
                        }
                      }
                      frame #1 {
                        n2207 = Unbundle(w3970) -> ("amps"=w3969:dbl, "volts"=w3968:dbl, "pf"=w3967:dbl)
                        n2208 = case shown="True" w3971 {
                          tunnel: w3978 -> [_ w4010]
                          tunnel: w3977 -> [_ w4017]
                          tunnel: w3976 -> [_ _]
                          tunnel: w3975 -> [_ _]
                          tunnel: w3974 -> [_ w4016]
                          tunnel: w3973 -> [_ w4015]
                          tunnel: w3972 -> [_ w3980]
                          tunnel: w3969 -> [_ w4012]
                          tunnel: w3968 -> [_ w4011]
                          tunnel: w3967 -> [_ w4009]
                          tunnel: w3966 -> [_ w4001]
                          frame False {
                          }
                          frame True {
                            n2209 = local read "TDMS LAB04-2"() -> (w4014:refnum<k34>)
                            n2210 = Build Array(w4011) -> (w4006:dbl[])
                            n2211 = Build Array(w4009) -> (w4005:dbl[])
                            n2212 = Build Array(w4016) -> (w4004:dbl[])
                            n2213 = Build Array(w4017) -> (w4003:dbl[])
                            n2214 = Build Array(w4012) -> (w4008:dbl[])
                            n2215 = Build Array(w4010) -> (w4007:dbl[])
                            n2216 = Build Array(w4015) -> (w4002:dbl[])
                            n2217 = Build Array("AMPS ON", "AMPS OFF", "VOLTS", "PF", "TEMP Live", "TEMP Neut", "CYCLE") -> (w3985:string[])
                            n2218 = Bundle By Name("Y"=w4008, "t0"=w4001) -> (w4000:waveform(dbl))  [unwired: 1 in]
                            n2219 = Bundle By Name("Y"=w4007, "t0"=w4001) -> (w3999:waveform(dbl))  [unwired: 1 in]
                            n2220 = Bundle By Name("Y"=w4006, "t0"=w4001) -> (w3998:waveform(dbl))  [unwired: 1 in]
                            n2221 = Bundle By Name("Y"=w4005, "t0"=w4001) -> (w3997:waveform(dbl))  [unwired: 1 in]
                            n2222 = Bundle By Name("Y"=w4004, "t0"=w4001) -> (w3996:waveform(dbl))  [unwired: 1 in]
                            n2223 = Bundle By Name("Y"=w4003, "t0"=w4001) -> (w3995:waveform(dbl))  [unwired: 1 in]
                            n2224 = Bundle By Name("Y"=w4002, "t0"=w4001) -> (w3994:waveform(dbl))  [unwired: 1 in]
                            n2225 = Build Array(w4000, w3999, w3998, w3997, w3996, w3995, w3994) -> (w3993:waveform(dbl)[])
                            n2226 = TDMS Write(0:w4014, 5:"TEST VALUES", 7:w3985, 9:w3993) -> (4:w3984:refnum<k34>, 6:w3983:string, 15:w3982:errorcluster)  [unwired: 2 in, 1 out]
                            n2227 = TDMS Write(0:w3984, 5:w3983, 7:"TIME", 9:w3980, 11:w3982) -> (15:w3979:errorcluster)  [unwired: 1 in, 3 out]
                            n2228 = local write "data file error"(w3979) -> ()
                          }
                        }
                      }
                    }
                  }
                }
              }
              frame #8 {
                n2229 = case shown="True" w4018 {
                  tunnel: w4022 -> [_ w4027]
                  tunnel: w4021 -> [_ w4026]
                  tunnel: w4020 -> [_ w4024]
                  tunnel: w4019 -> [_ w4023]
                  frame False {
                  }
                  frame True {
                    n2230 = local read "DISP LAB05-1"() -> (w4028:T4)
                    n2231 = local read "SIG LAB05-1"() -> (w4029:T2)
                    n2232 = local read "ON L05-1"() -> (w4025:cluster{"amps":dbl, "volts":dbl, "pf":dbl})
                    n2233 = Unbundle(w4029) -> ("AMPS"=w4035:dbl, "VOLTS"=w4033:dbl, "PF"=w4032:dbl, "Tmp Live"=w4031:dbl, "Tmp Neut"=w4034:dbl)
                    n2234 = Unbundle(w4028) -> ("CYCLE"=w4030:dbl)  [unwired: 2 out]
                    n2235 = stacked-sequence {
                      tunnel: w4035 -> [w4039 w4058]
                      tunnel: w4034 -> [_ w4057]
                      tunnel: w4033 -> [w4038 w4056]
                      tunnel: w4032 -> [w4037 w4055]
                      tunnel: w4031 -> [_ w4054]
                      tunnel: w4030 -> [_ w4053]
                      tunnel: w4027 -> [_ w4052]
                      tunnel: w4026 -> [w4040 _]
                      tunnel: w4025 -> [w4036 w4050]
                      tunnel: w4024 -> [_ w4051]
                      tunnel: w4023 -> [_ w4046]
                      frame #0 {
                        n2236 = case shown="True" w4040 {
                          tunnel: w4039 -> [_ w4045]
                          tunnel: w4038 -> [_ w4044]
                          tunnel: w4037 -> [_ w4043]
                          tunnel: w4036 -> [_ w4041]
                          frame False {
                          }
